vi "Boiler room KKK.vi"() -> ()   [LabVIEW 2023]
panel:
  in  "min temp":dbl=20.0
  in  "max temp":dbl=80.0
  in  "Automatic / Manual":bool
  out "Thermometer":dbl(slide) scale=0.0..100.0
  out "AC":bool
  out "Heater":bool
  out "Manual":bool
  in  "Heater":bool
  in  "AC":bool
  in  "stop":bool
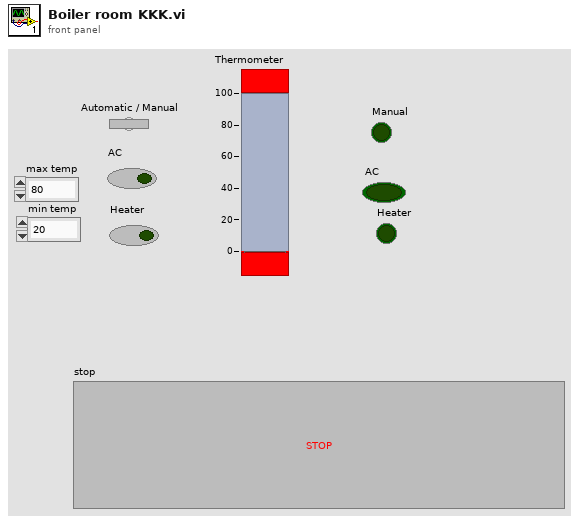
[diagram p1: front panel]
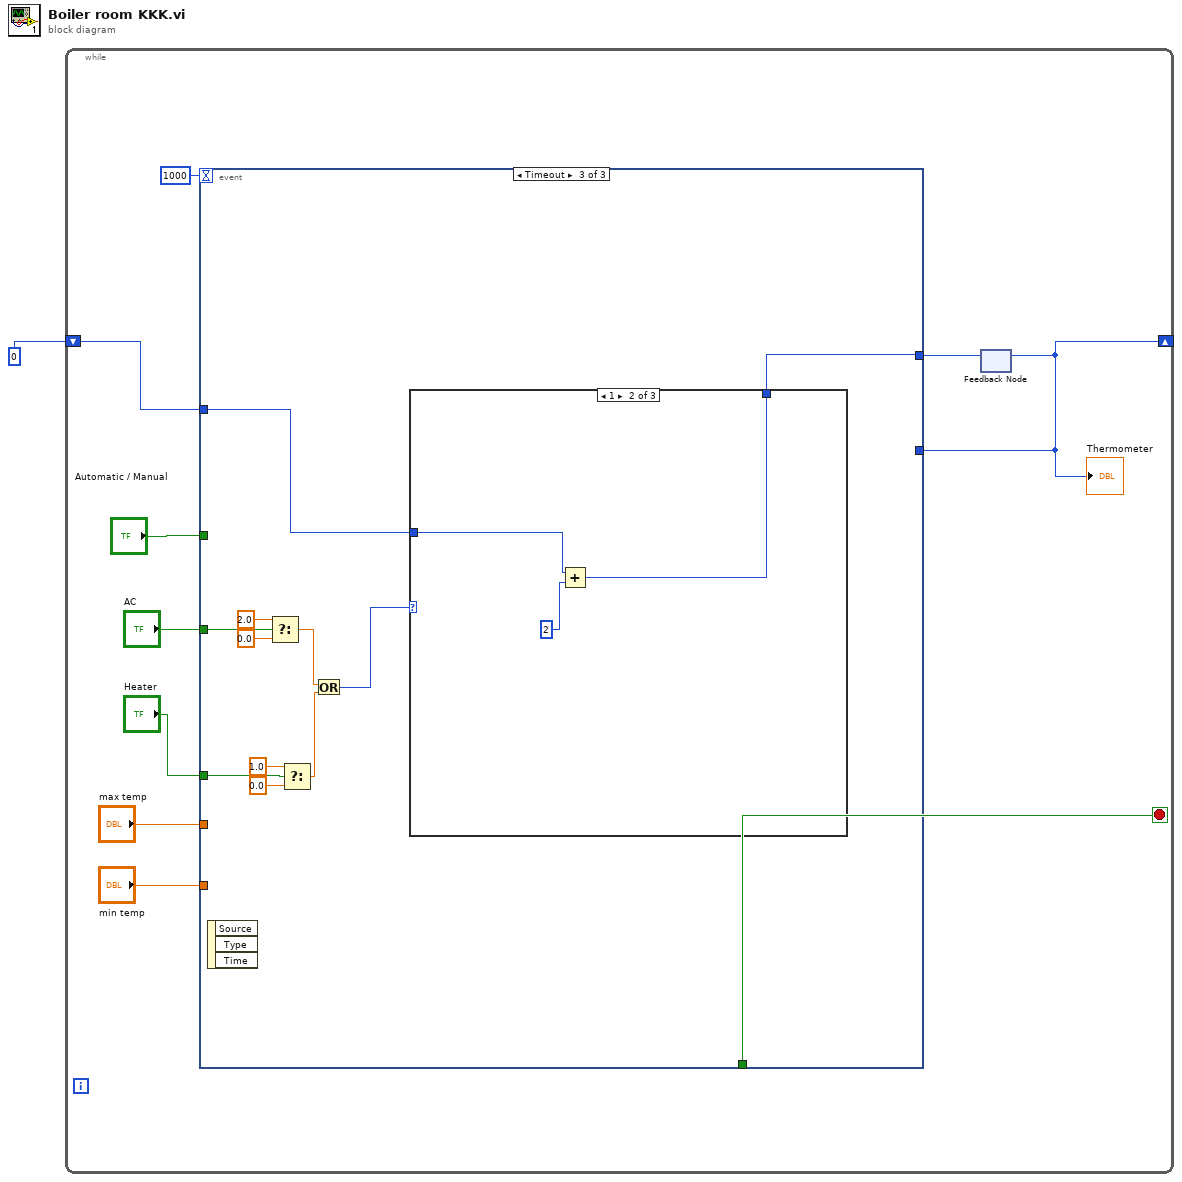
[diagram p0: block diagram]
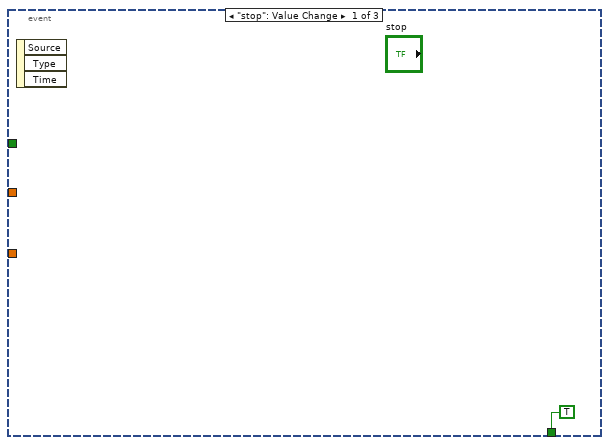
[diagram p2: hidden frame]
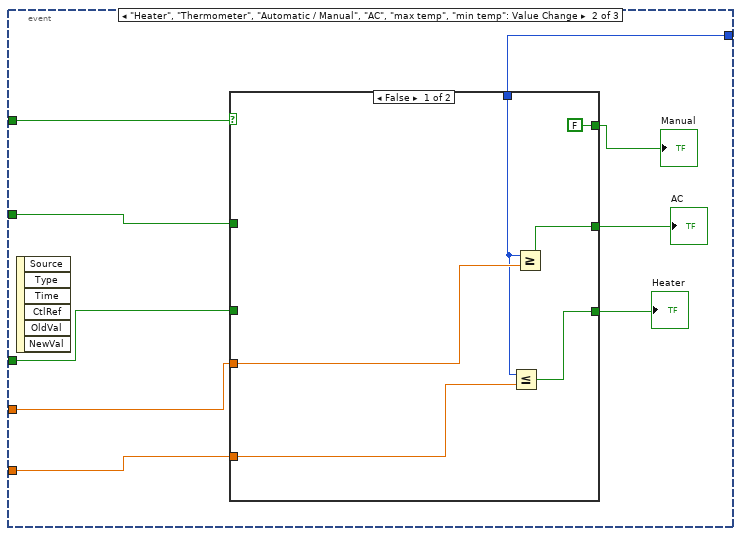
[diagram p3: hidden frame]
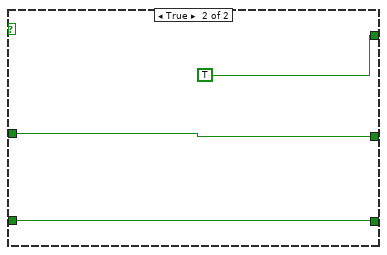
[diagram p4: hidden frame]
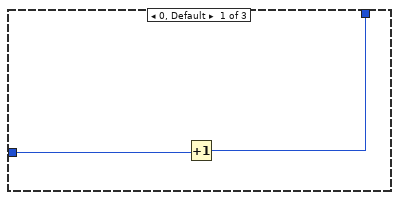
[diagram p5: hidden frame]
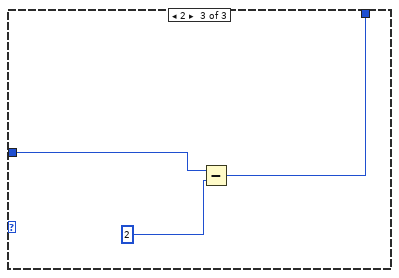
[diagram p6: hidden frame]
diagram:
  n1 = while {
    shift-right: [w2] -> _
    shift-left: 0 -> [w9]
    stop <- w11 stop-if-true
    n2 = feedback #1() -> (w2:i32)  [unwired: 1 in]
    "Thermometer" <- w2
    n3 = event shown="[2] Timeout" {
      selector: _ -> [_ _ _]
      dyn-events: _ -> [_ _ _]
      timeout: 1000 -> [_ _ _]
      tunnel: [TRUE _ _] -> w11
      tunnel: w9 -> [_ _ w35]
      tunnel: "Automatic / Manual" -> [_ w21 _]
      tunnel: "AC" -> [_ w20 w40]
      tunnel: "Heater" -> [_ w19 w41]
      tunnel: "max temp" -> [_ w18 _]
      tunnel: "min temp" -> [_ w17 _]
      tunnel: [_ _ w31] -> w3
      tunnel: w2 -> [_ w13 _]
      event "stop": Value Change {
        n4 = event-data() -> ()  [unwired: 1 in, 3 out]
      }
      event "Heater", "Thermometer", "Automatic / Manual", "AC", "max temp", "min temp": Value Change {
        n5 = event-data() -> ()  [unwired: 1 in, 6 out]
        n6 = case shown="False" w21 {
          tunnel: [w26 w30] -> w14
          tunnel: w19 -> [_ w30]
          tunnel: [w27 w29] -> w15
          tunnel: w20 -> [_ w29]
          tunnel: [FALSE TRUE] -> w16
          tunnel: w18 -> [w24 _]
          tunnel: w17 -> [w23 _]
          tunnel: w13 -> [w22 _]
          frame False {
            n7 = Less Or Equal?(x=w22, y=w23) -> (x <= y?=w26:bool)
            n8 = Greater Or Equal?(x=w22, y=w24) -> (x >= y?=w27:bool)
          }
          frame True {
          }
        }
        "Manual" <- w16
        "AC" <- w15
        "Heater" <- w14
      }
      event Timeout {
        n9 = event-data() -> ()  [unwired: 1 in, 3 out]
        n10 = Select(t=2.0, s=w40, f=0.0) -> (s? t:f=w33:dbl)
        n11 = Select(t=1.0, s=w41, f=0.0) -> (s? t:f=w34:dbl)
        n12 = Or(x=w33, y=w34) -> (x .or. y?=w32:i32)
        n13 = case shown="1" w32 {
          tunnel: w35 -> [w43 w46 w49]
          tunnel: [w42 w44 w47] -> w31
          frame 0, Default {
            n14 = Increment(x=w43) -> (x+1=w42:i32)
          }
          frame 1 {
            n15 = Add(x=w46, y=2) -> (x+y=w44:i32)
          }
          frame 2 {
            n16 = Subtract(x=w49, y=2) -> (x-y=w47:i32)
          }
        }
      }
    }
    n17 = feedback-in #1(w3) -> ()
  }
